vi "Write Encryption.vi"(10 "Encryption":refnum<class "Encryption.lvclass">, 11 "ConfigManager in":refnum<class "ConfigManager.lvclass">) -> (3 "ConfigManager out":refnum<class "ConfigManager.lvclass">)   [LabVIEW 2013, in "CfgManager.lvlib" / "ConfigManager.lvclass"]
uses:
  ConfigManager.lvclass
  Encryption/Encryption.lvclass
  ConfigManager.lvclass/ConfigManager.ctl
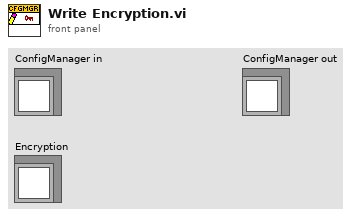
[diagram p1: front panel]
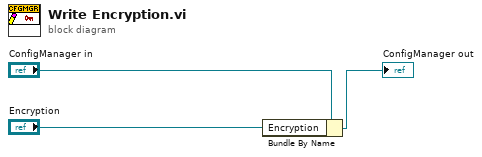
[diagram p0: block diagram]
diagram:
  n1 = Bundle By Name(cluster="ConfigManager in", "Encryption"="Encryption") -> (→"ConfigManager out":refnum<class "ConfigManager.lvclass">)
